vi "Swerve Wheel.vi"(7 "Wheel":T1(ring), 10 "Inputs":dbl[](array[numeric])) -> (1 "Speed":dbl, 2 "Motor Output":dbl)   [LabVIEW 2017]
uses:
  Public/Documents/Cross The Road Electronics/Phoenix-LabVIEW/Motor Controller/Controls/CTRE_Phoenix_MotorControl_ControlMode.ctl
  <vilib>/Rock Robotics/Network Tables/NT Read Number.vi
  <vilib>/Rock Robotics/Network Tables/NT Write Number.vi
  <vilib>/addons/control/pid/pid.llb/PID (DBL).vi
  <vilib>/addons/control/pid/NI_PID_pid.lvlib
panel:
  out "PID Values":cluster{"P":dbl, "I":dbl, "D":dbl}
  # "Swerve Wheel Control\nFRC Team 34"
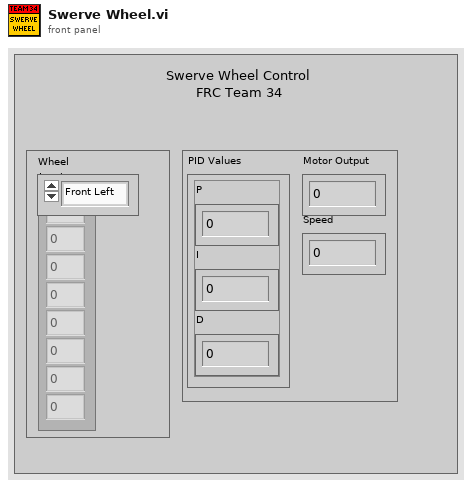
[diagram p1: front panel]
types:
  T1 = enum16{"Front Left", "Front Right", "Back Left", "Back Right"}
  T2 = typedef "CTRE_Phoenix_MotorControl_ControlMode.ctl" = u16
  T3 = enum16{"Z", "Y", "X", "Rot. Point X", "Rot. Point Y", "Width/2", "Max", "Length/2"}
  T4 = enum16{"Z Axis", "Y", "X", "Rot. Point X", "Rot. Point Y", "Width/2", "Max", "Length/2"}
  T5 = typedef "WPI_MotorControlDeviceRef.ctl" = cluster{"DeviceStatus":errorcluster, "Type":T6, "PWM":cluster{"PWM Channel":T7, "DeadBand":T8}, "CAN":cluster{"Device Number":u8, "SetOutput VI Ref":variant, "GetOutput VI Ref":variant, "Enable VI Ref":variant, "Disable VI Ref":variant, "Data":variant}, "Invert":bool, "DIO PWM":cluster{"PWM \"Enable\" Channel":T7, "DIOChannel":T9, "PWM Rate":dbl}}
  T6 = typedef "WPI_MotorControlType.ctl" = enum16{"PWM", "CAN", "DIO PWM"}
  T7 = typedef "FPGA_DIOPWMChannel.ctl" = enum8{"PWM 0", "PWM 1", "PWM 2", "PWM 3", "PWM 4", "PWM 5", "PWM 6", "PWM 7", "PWM 8", "PWM 9", "PWM MXP 0", "PWM MXP 1", "PWM MXP 2", "PWM MXP 3", "PWM MXP 4", "PWM MXP 5", "PWM MXP 6", "PWM MXP 7", "PWM MXP 8", "PWM MXP 9", "Invalid"}
  T8 = typedef "WPI_PWMDeadband.ctl" = cluster{"Name":string, "maxPositivePwm":i32, "minPositivePwm":i32, "centerPwm":i32, "maxNegativePwm":i32, "minNegativePwm":i32, "angularRange":u16}
  T9 = typedef "FPGA_DIOChannel.ctl" = enum8{"DIO 0", "DIO 1", "DIO 2", "DIO 3", "DIO 4", "DIO 5", "DIO 6", "DIO 7", "DIO 8", "DIO 9", "DIO MXP 0", "DIO MXP 1", "DIO MXP 2", "DIO MXP 3", "DIO MXP 4", "DIO MXP 5", "DIO MXP 6", "DIO MXP 7", "DIO MXP 8", "DIO MXP 9", "DIO MXP 10", "DIO MXP 11", "DIO MXP 12", "DIO MXP 13", "DIO MXP 14", "DIO MXP 15", "SPI Port CS1", "SPI Port CS2", "SPI Port CS3", "SPI Port MISO", "SPI Port MOSI", "Invalid"}
  T10 = typedef "WPI_EncoderDevRef.ctl" = cluster{"DevStatus":errorcluster, "EncoderIndex":T11, "CounterIndex":T12, "DistancePerCount":dbl, "Decoding Type":T13}
  T11 = typedef "FPGA_EncoderIdx.ctl" = enum8{"Enc 0", "Enc 1", "Enc 2", "Enc 3", "Enc 4", "Enc 5", "Enc 6", "Enc 7", "Invalid"}
  T12 = typedef "FPGA_CounterCtrSystemIndex.ctl" = enum8{"Ctr 0", "Ctr 1", "Ctr 2", "Ctr 3", "Ctr 4", "Ctr 5", "Ctr 6", "Ctr 7", "Invalid"}
  T13 = typedef "WPI_EncoderType.ctl" = enum16{"1x", "2x", "4x"}
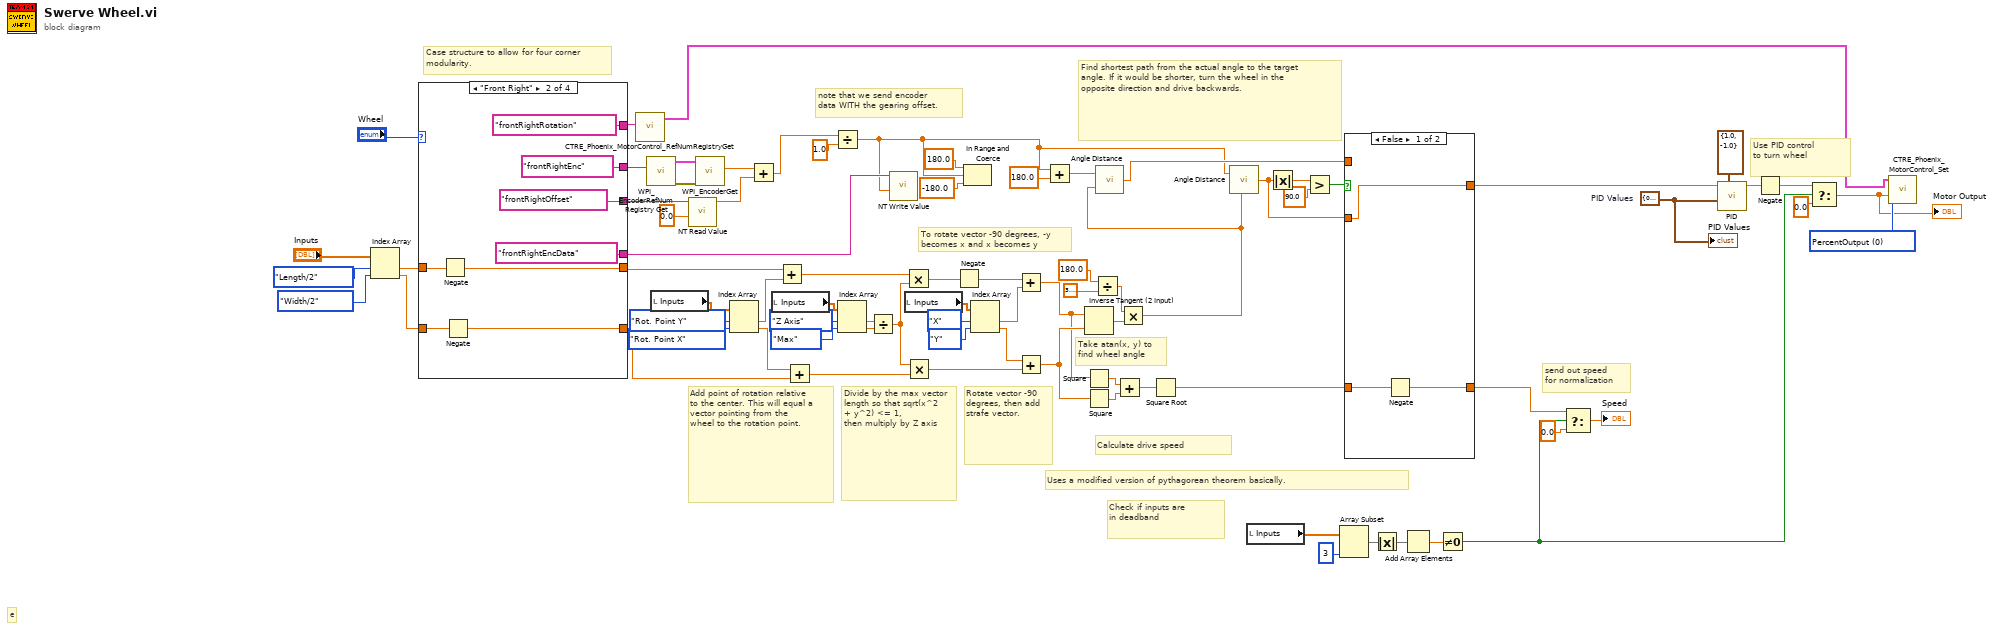
[diagram p0: block diagram]
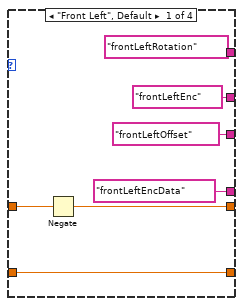
[diagram p3: hidden frame]
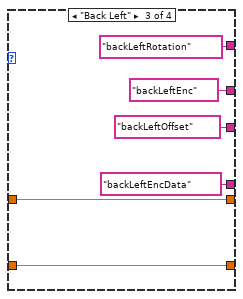
[diagram p4: hidden frame]
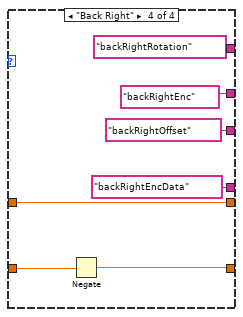
[diagram p5: hidden frame]
diagram:
  w2 = T2 0 items=["PercentOutput"=0, "Position"=1, "Velocity"=2, "Current"=3, "Follower"=5, "MotionProfile"=6, "MotionMagic"=7, "MotionMagicArc"=8, "MotionProfileArc"=10, "Disabled"=15] ("Control Mode")
  w5 = cluster{"P":dbl, "I":dbl, "D":dbl} {"P"=0.1, "I"=0.0, "D"=0.0}  # PID Values
  # "Uses a modified version of pythagorean theorem basically."
  # "e"
  # "note that we send encoder \ndata WITH the gearing offset."
  # "Case structure to allow for four corner\nmodularity."
  # "To rotate vector -90 degrees, -y becomes x and x becomes y"
  # "send out speed\nfor normalization"
  # "Use PID control\nto turn wheel"
  # "Find shortest path from the actual angle to the target angle. If it would be shorter, turn the wheel in the opposite direction and drive backwards."
  # "Divide by the max vector length so that sqrt(x^2 + y^2) <= 1,\nthen multiply by Z axis"
  # "Add point of rotation relative to the center. This will equal a vector pointing from the\nwheel to the rotation point."
  # "Check if inputs are\nin deadband"
  # "Take atan(x, y) to find wheel angle"
  # "Calculate drive speed"
  # "Rotate vector -90 degrees, then add strafe vector."
  n1 = Index Array(array="Inputs", index #1=T3."Length/2", index #2=T3."Width/2") -> (element #1=w75:dbl, element #2=w74:dbl)
  n2 = case shown="\"Front Right\"" "Wheel" {
    tunnel: w75 -> [w86 w94 w100 w107]
    tunnel: w74 -> [w84 w92 w99 w106]
    tunnel: [w85 w93 w100 w107] -> w43
    tunnel: [w84 w91 w99 w105] -> w42
    tunnel: ["frontLeftRotation" "frontRightRotation" "backLeftRotation" "backRightRotation"] -> w4
    tunnel: ["frontLeftEnc" ("refnum name") "frontRightEnc" ("refnum name") "backLeftEnc" ("refnum name") "backRightEnc" ("refnum name")] -> w55
    tunnel: ["frontLeftOffset" ("Name") "frontRightOffset" ("Name") "backLeftOffset" ("Name") "backRightOffset" ("Name")] -> w51
    tunnel: ["frontLeftEncData" ("Name") "frontRightEncData" ("Name") "backLeftEncData" ("Name") "backRightEncData" ("Name")] -> w12
    frame "Front Left", Default {
      n3 = Negate(x=w86) -> (-x=w85:dbl)
    }
    frame "Front Right" {
      n4 = Negate(x=w94) -> (-x=w93:dbl)
      n5 = Negate(x=w92) -> (-x=w91:dbl)
    }
    frame "Back Left" {
    }
    frame "Back Right" {
      n6 = Negate(x=w106) -> (-x=w105:dbl)
    }
  }
  n7 = call "CTRE_Phoenix_MotorControl_RefNumRegistryGet.vi"("refnum name"=w4) -> ("PhoenixMotorControlDevRef"=w3:T5)  [unwired: 9 in, 1 out]
  n8 = call <vilib>:"WPI_EncoderRefNum Registry Get.vi"("refnum name"=w55) -> ("error out"=w54:errorcluster, "EncoderDevRef"=w53:T10)  [unwired: 9 in]
  n9 = local read "Inputs"() -> (w48:dbl[])
  n10 = call-poly <vilib>:"NT Read Value.vi"("Default Value"=0.0, "Name"=w51) -> ("Numeric"=w46:dbl)  [unwired: 8 in, 1 out]
  n11 = call <vilib>:"WPI_EncoderGet.vi"("error in (no error)"=w54, "EncoderDevRef"=w53) -> ("Distance"=w47:dbl)  [unwired: 4 in, 5 out]
  n12 = Index Array(array=w48, index #1=T3."Rot. Point Y", index #2=T3."Rot. Point X") -> (element #1=w44:dbl, element #2=w45:dbl)
  n13 = Add(x=w47, y=w46) -> (x+y=w11:dbl)
  n14 = local read "Inputs"() -> (w56:dbl[])
  n15 = Add(x=w43, y=w44) -> (x+y=w41:dbl)
  n16 = Add(x=w45, y=w42) -> (x+y=w66:dbl)
  n17 = Divide(x=w11, y=1.0) -> (x/y=w9:dbl)
  n18 = Index Array(array=w56, index #1=T4."Z Axis", index #2=T3."Max") -> (element #1=w14:dbl, element #2=w13:dbl)
  n19 = Divide(x=w14, y=w13) -> (x/y=w65:dbl)
  n20 = call-poly <vilib>:"NT Write Value.vi"("Numeric"=w9, "Name"=w12) -> ()  [unwired: 9 in, 1 out]
  n21 = Multiply(x=w41, y=w65) -> (x*y=w58:dbl)
  n22 = local read "Inputs"() -> (w17:dbl[])
  n23 = Multiply(x=w65, y=w66) -> (x*y=w61:dbl)
  n24 = Negate(x=w58) -> (-x=w57:dbl)
  n25 = In Range and Coerce(upper limit=180.0, x=w9, lower limit=-180.0 ("upper limit")) -> ()  [unwired: 2 out]
  n26 = Index Array(array=w17, index #1=T3."X", index #2=T3."Y") -> (element #1=w16:dbl, element #2=w15:dbl)
  n27 = Add(x=w57, y=w16) -> (x+y=w59:dbl)
  n28 = Add(x=w15, y=w61) -> (x+y=w60:dbl)
  n29 = Add(x=w9, y=180.0) -> (x+y=w38:dbl)
  n30 = Inverse Tangent (2 Input)(1:w60, 2:w59) -> (0:w73:dbl)
  n31 = Square(x=w59) -> (x^2=w62:dbl)
  n32 = Square(x=w60) -> (x^2=w72:dbl)
  n33 = Divide(x=180.0 ("y"), y=3.141592653589793) -> (x/y=w70:dbl)
  n34 = Add(x=w62, y=w72) -> (x+y=w71:dbl)
  n35 = Multiply(x=w70, y=w73) -> (x*y=w39:dbl)
  n36 = call "Angle Distance.vi"("Target Angle"=w39, "Current Angle"=w38) -> ("Distance"=w31:dbl)
  n37 = Square Root(x=w71) -> (sqrt(x)=w33:dbl)
  n38 = call "Angle Distance.vi"("Target Angle"=w39, "Current Angle"=w9) -> ("Distance"=w32:dbl)
  n39 = local read "Inputs"() -> (w27:dbl[])
  n40 = Absolute Value(x=w32) -> (abs(x)=w36:dbl)
  n41 = Greater?(x=w36, y=90.0) -> (0:w34:bool)
  n42 = Array Subset(array=w27, length=3) -> (w29:dbl[])  [unwired: 1 in]
  n43 = case shown="False" w34 {
    tunnel: w33 -> [w109 w111]
    tunnel: w32 -> [w110 _]
    tunnel: w31 -> [_ w112]
    tunnel: [w108 w111] -> w25
    tunnel: [w110 w112] -> w6
    frame False {
      n44 = Negate(x=w109) -> (-x=w108:dbl)
    }
    frame True {
    }
  }
  n45 = Absolute Value(x=w29) -> (abs(x)=w28:dbl[])
  n46 = Add Array Elements(numeric array=w28) -> (sum=w30:dbl)
  n47 = Not Equal To 0?(x=w30) -> (x != 0?=w18:bool)
  n48 = Select(t=w25, s=w18, f=0.0) -> (s? t:f=→"Speed":dbl)
  n49 = call-poly <vilib>:"PID.vi"("output range"=cluster{"output high":dbl, "output low":dbl} {"output high"=1.0, "output low"=-1.0}, "PID gains"=w5, "setpoint"=w6) -> ("output"=w21:dbl)  [unwired: 7 in, 1 out]
  n50 = Negate(x=w21) -> (-x=w19:dbl)
  n51 = Select(t=w19, s=w18, f=0.0) -> (s? t:f=w1:dbl)
  "Motor Output" <- w1
  n52 = call "CTRE_Phoenix_MotorControl_Set.vi"("Output"=w1, "Control Mode"=w2, "PhoenixMotorControlDevRef"=w3) -> ()  [unwired: 6 in, 3 out]
  "PID Values" <- w5
